vi "Find Value Indexies.vi"(10 "Value":i32, 11 "Array":i32[](array[numeric])) -> (3 "Value indexies":i32[](array[numeric]))   [LabVIEW 2016]
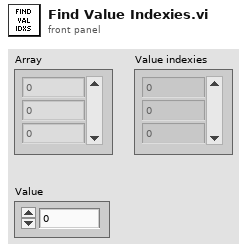
[diagram p1: front panel]
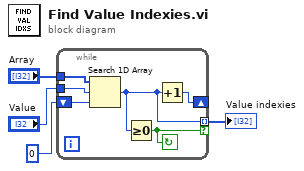
[diagram p0: block diagram]
diagram:
  n1 = while {
    tunnel: "Array" -> [w10]
    tunnel: "Value" -> [w9]
    shift-right: [w5] -> _
    shift-left: 0 ("start index (0)") -> [w8]
    tunnel: [w6] -> w1 mode=indexing if=w7
    stop <- w7 continue-if-true
    n2 = Search 1D Array(1D array=w10, element=w9, start index (0)=w8) -> (index of element=w6:i32)
    n3 = Greater Or Equal To 0?(x=w6) -> (x >= 0?=w7:bool)
    n4 = Increment(x=w6) -> (x+1=w5:i32)
  }
  "Value indexies" <- w1
